vi "example_3_5_a.vi"() -> ()   [LabVIEW 2018]
panel:
  out "Response":string
  # "NOTE: remember plug the Led Analyser\nbefore run LabVIEW and to change the\nVISA resource name in the schematic,\notherwise the application will not work."
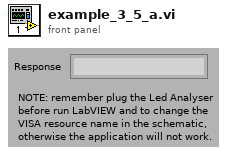
[diagram p1: front panel]
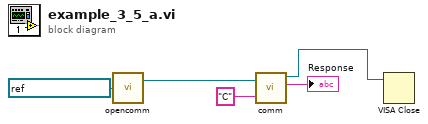
[diagram p0: block diagram]
diagram:
  n1 = call "opencomm.vi"("VISA resource name"=refnum<visa-resource-name> "ASRL20::INSTR") -> ("duplicate VISA resource name"=w4:refnum<visa-resource-name>)  [unwired: 1 out]
  n2 = call "comm.vi"("VISA resource name"=w4, "Command"="C") -> ("dup VISA resource name"=w2:refnum<visa-resource-name>, "Response"=→"Response":string)  [unwired: 2 out]
  n3 = VISA Close(VISA resource name=w2) -> ()  [unwired: 1 in, 1 out]
